vi "两点之间距离.vi"(8 "Error In":errorcluster caption="错误输入", 10 "点B":T1, 11 "点A":T1) -> (0 "Error Out":errorcluster caption="错误输出", 3 "距离AB":dbl)   [LabVIEW 2012, in "几何工具.lvlib"]
uses:
  <vilib>/Utility/miscctls.llb/LVPointDoubleTypeDef.ctl
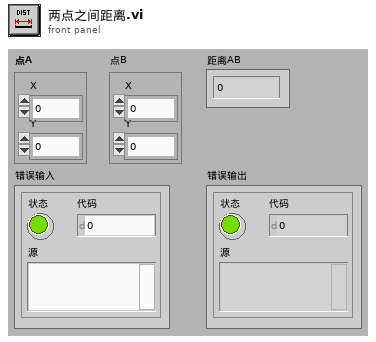
[diagram p1: front panel]
types:
  T1 = typedef "LVPointDoubleTypeDef.ctl" = cluster{"X":dbl, "Y":dbl}
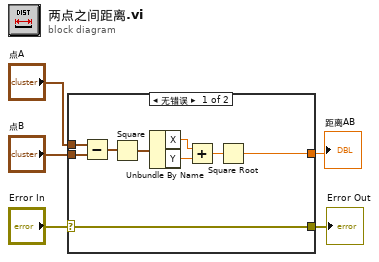
[diagram p0: block diagram]
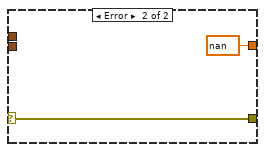
[diagram p2: hidden frame]
diagram:
  n1 = case shown="无错误" "Error In" {
    selector: "Error In" -> [w11 w16]
    tunnel: "点A" -> [w13 _]
    tunnel: "点B" -> [w12 _]
    tunnel: [w11 w16] -> w2
    tunnel: [w6 nan] -> w1
    frame No Error {
      n2 = Subtract(x=w13, y=w12) -> (x-y=w14:T1)
      n3 = Square(x=w14) -> (x^2=w10:T1)
      n4 = Unbundle By Name(w10) -> ("X"=w8:dbl, "Y"=w9:dbl)
      n5 = Add(x=w8, y=w9) -> (x+y=w7:dbl)
      n6 = Square Root(x=w7) -> (sqrt(x)=w6:dbl)
    }
    frame Error {
    }
  }
  "Error Out" <- w2
  "距离AB" <- w1
